vi "Trigger Detection for N Channel.vi"(0 "signal in":waveform(dbl)[](array[waveform]), 1 "reset":bool, 5 "level":dbl[](array[numeric]) format="%0.2f", 7 "hysteresis":dbl[](array[numeric]) format="%0.2f", 9 "location mode":u16(ring) items=["Index", "Time"], 11 "error in (no error)":errorcluster, 12 "trigger slope":u16[](array[ring]) items=["Falling Edge", "Rising Edge"]) -> (4 "trigger locations":dbl[](array[numeric]) format="%#.2g", 6 "trigger detected?":bool[](array[boolean]), 15 "error out":errorcluster)   [LabVIEW 2020, in "NI_MAPro.lvlib"]
doc: "Finds the first level-crossing location in a waveform. You can retrieve the trigger location as an index or as a time. The trigger conditions are specified in terms of threshold <B>level</B>, <B>slope</B>, and <B>hysteresis</B>. Wire data to the <B>signal in</B> input to determine the polymorphic instance to use or manually select the instance."
uses:
  NI_MAPro.lvlib
  NI_MABase.lvlib
  <resource>/lvanlys.dll
panel:
  out "number of triggers detected":i32[](array[numeric])
  out "triggerDetectedbyte":i32[](array[numeric])
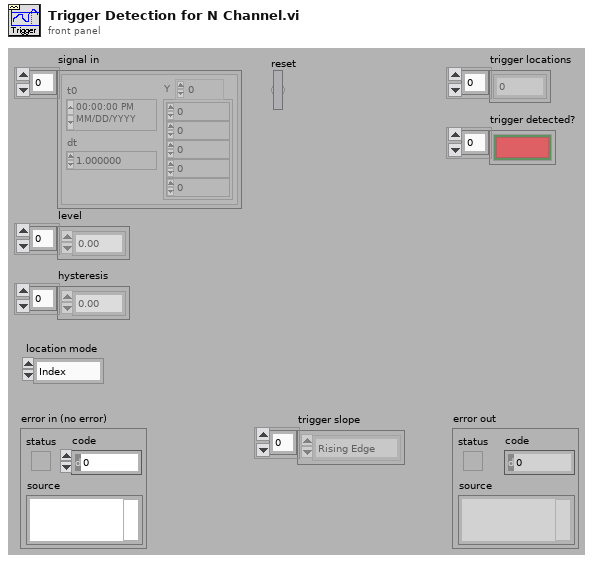
[diagram p1: front panel]
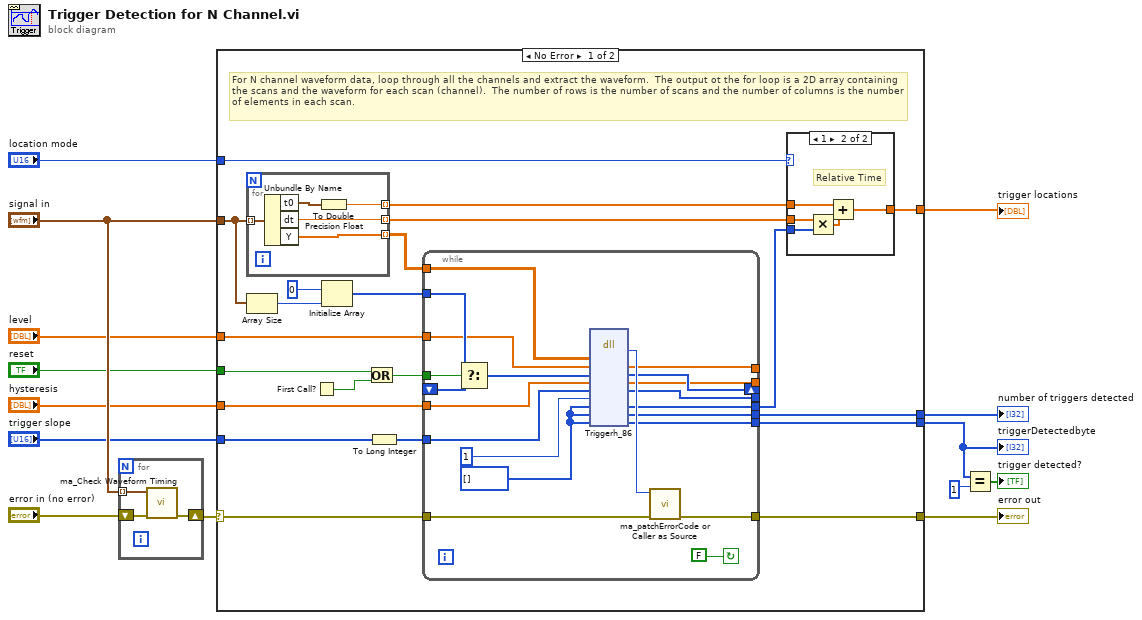
[diagram p0: block diagram]
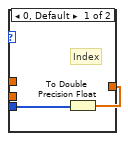
[diagram p2: hidden frame]
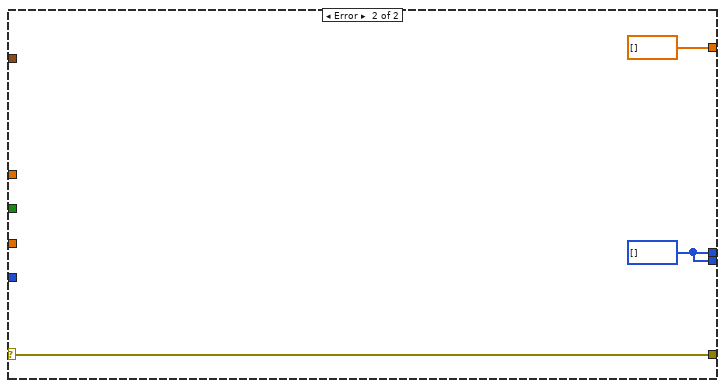
[diagram p3: hidden frame]
diagram:
  n1 = for {
    tunnel: "signal in" -> [w15] mode=indexing
    shift-right: [w16] -> w4
    shift-left: "error in (no error)" -> [w17]
    n2 = call "ma_Check Waveform Timing.vi"("error in (no error)"=w17, "signal in"=w15) -> ("error out"=w16:errorcluster)  [unwired: 1 in, 8 out]
  }
  n3 = case shown="No Error" w4 {
    selector: w4 -> [w38 w74]
    tunnel: [w37 w74] -> w13
    tunnel: "signal in" -> [w21 _]
    tunnel: "reset" -> [w34 _]
    tunnel: "trigger slope" -> [w19 _]
    tunnel: "hysteresis" -> [w36 _]
    tunnel: "level" -> [w29 _]
    tunnel: [w25 dbl[] []] -> w8
    tunnel: "location mode" -> [w20 _]
    tunnel: [w28 w73] -> w3
    tunnel: [w27 w73] -> w2
    frame No Error {
      # "For N channel waveform data, loop through all the channels and extract the waveform.  The output ot the for loop is a 2D array containing the scans and the waveform for each scan (channel).  The number of rows is the number of scans and the number of columns is the number of elements in each scan."
      n4 = for {
        tunnel: [w50] -> w26 mode=indexing
        tunnel: [w47] -> w22 mode=indexing
        tunnel: [w49] -> w24 mode=indexing
        tunnel: w21 -> [w46] mode=indexing
        n5 = Unbundle By Name(w46) -> ("t0"=w48:timestamp, "dt"=w47:dbl, "Y"=w50:dbl[])
        n6 = To Double Precision Float(number=w48) -> (double precision float=w49:dbl)
      }
      n7 = Array Size(array=w21) -> (size(s)=w31:i32)
      n8 = First Call?() -> (First Call?: T/F=w35:bool)
      n9 = Initialize Array(0, w31) -> (w30:i32[])
      n10 = Or(x=w34, y=w35) -> (x .or. y?=w33:bool)
      n11 = To Long Integer(number=w19) -> (32bit integer=w18:i32[])
      n12 = while {
        tunnel: w38 -> [w55]
        tunnel: [w54] -> w37
        shift-right: [w67] -> _
        shift-left: _ -> [w70]
        tunnel: w18 -> [w66]
        tunnel: w36 -> [w65]
        tunnel: w33 -> [w64]
        tunnel: w30 -> [w63]
        tunnel: w29 -> [w62]
        tunnel: [w61] -> w28
        tunnel: [w60] -> w27
        tunnel: w26 -> [w59]
        tunnel: [w58] -> w23
        tunnel: [w53] -> _
        tunnel: [w52] -> _
        tunnel: [w51] -> _
        stop <- FALSE continue-if-true
        w56 = i32[] [] ("Array Constant")
        n13 = Select(t=w63, s=w64, f=w70) -> (s? t:f=w69:i32[])
        n14 = dll-call lib="C:/Program Files (x86)/National Instruments/LabVIEW 2020/resource/lvanlys.*" fn="Triggerh_86"("x"=w59, "level"=w62, "status"=w69, "hysterisis"=w65, "slope"=w66, "ntptsH"=1 ("max number trigger pts"), "triggerIndex"=w56, "number_of_triggers_detected"=w56, "triggerDetectedbyte"=w56) -> ("return type"=w71:i32, "level"=w53:dbl[], "status"=w67:i32[], "hysterisis"=w52:dbl[], "slope"=w51:i32[], "triggerIndex"=w58:i32[], "number_of_triggers_detected"=w61:i32[], "triggerDetectedbyte"=w60:i32[])  [unwired: 5 in, 2 out]
        n15 = call "ma_patchErrorCode or Caller as Source.vi"("error in (no error)"=w55, "error code"=w71) -> ("error out"=w54:errorcluster)  [unwired: 2 in, 7 out]
      }
      n16 = case shown="1" w20 {
        tunnel: w23 -> [w40 w45]
        tunnel: [w39 w42] -> w25
        tunnel: w22 -> [_ w44]
        tunnel: w24 -> [_ w41]
        frame 0, Default {
          # "Index"
          n17 = To Double Precision Float(number=w40) -> (double precision float=w39:dbl[])
        }
        frame 1 {
          # "Relative Time"
          n18 = Multiply(x=w44, y=w45) -> (x*y=w43:dbl[])
          n19 = Add(x=w41, y=w43) -> (x+y=w42:dbl[])
        }
      }
    }
    frame Error {
      w73 = i32[] [] ("number_of_triggers_detected")
    }
  }
  "error out" <- w13
  "trigger locations" <- w8
  "number of triggers detected" <- w3
  "triggerDetectedbyte" <- w2
  n20 = Equal?(x=w2, y=1 ("Element Data")) -> (x = y?=→"trigger detected?":bool[])
